vi "Measurement.vi"() -> ()   [LabVIEW 2015]
doc: "Use this template to build a producer/consumer design pattern with events to produce queue items. Use this design pattern instead of the User Interface Event Handler pattern for user interfaces when you want to execute code asynchronously in response to an event without slowing the user interface responsiveness."
uses:
  C:/Program Files (x86)/National Instruments/LabVIEW 2015/examples/Data Communication/Protocols/TCP/TCP Multiple Connections/controls/TCP Multiple Connections State.ctl
panel:
  out "Number  of dev Connected":i32
  in  "Restart":bool
  out "IP Address":string
  out "Waveform_main 2":waveform(sgl)(graph)
  out "CT2":timestamp
  out "USB_DEV2":string
  out "USB_DEV1":string
  out "CT1":timestamp
  out "Waveform_main":waveform(sgl)(graph)
  # "uPower Server V1.0"
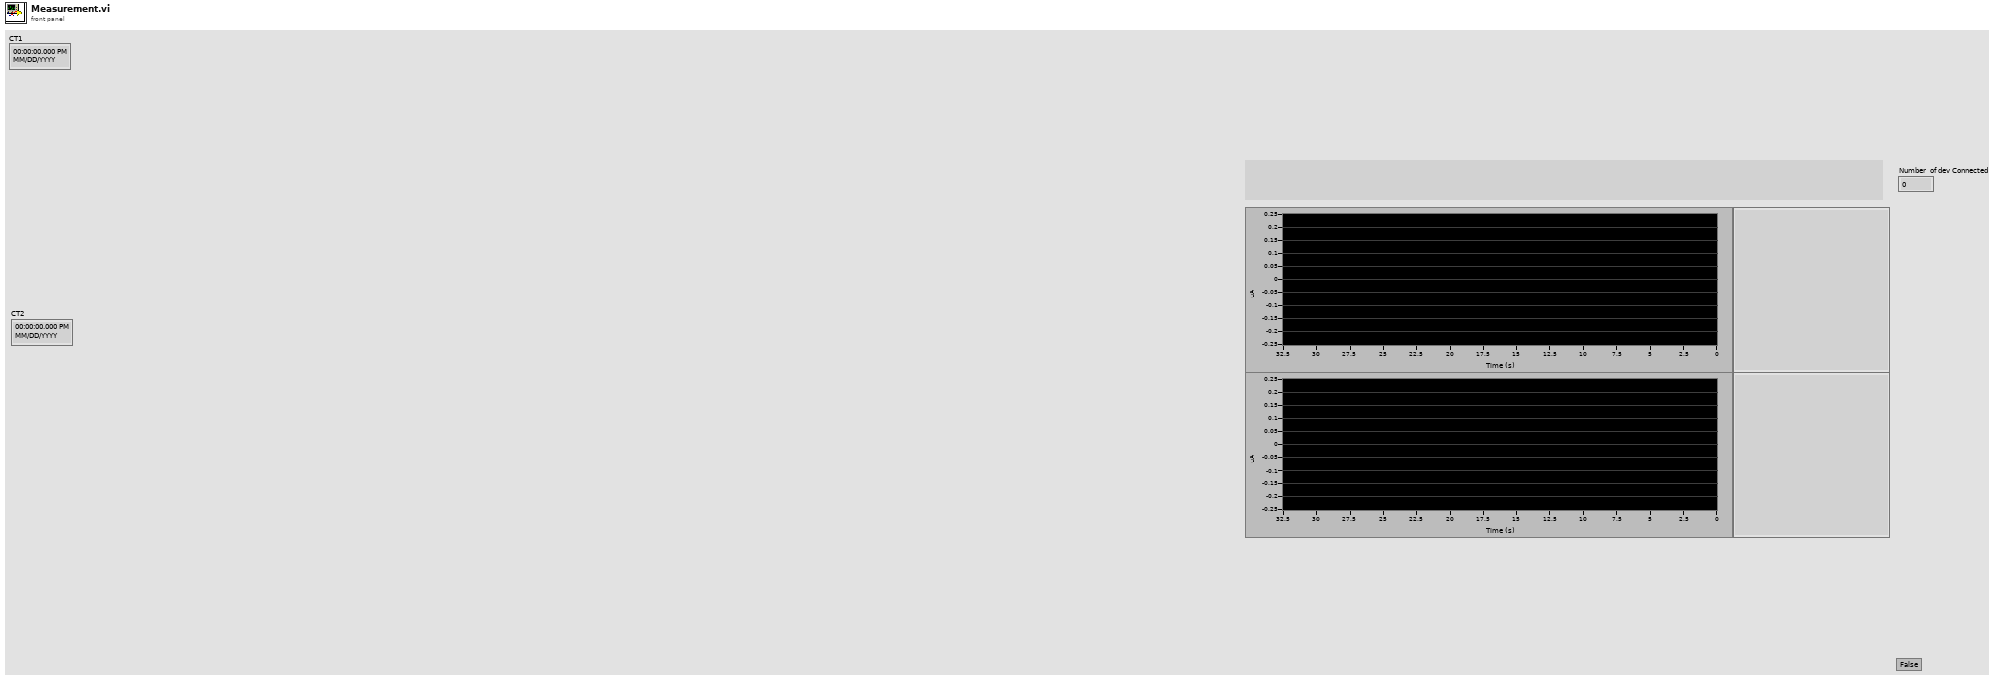
[diagram p1: front panel]
types:
  T1 = typedef "TCP Multiple Connections State.ctl" = enum16{"Initialize", "Status Check", "Measurement", "Return Values to DEV", "Stop"}
  T2 = typedef "uPower_kit.ctl" = cluster{"DEV":string, "BUSY":bool, "VBAT":dbl, "OUTPUT":bool, "LAST_RESULT":dbl, "DURATION":u16, "TRIGGER":bool, "RANGE":string, "Vsource":dbl, "FW":string, "Mode":string}
  T3 = typedef "imagedata.ctl" = cluster{"image type":i32, "image depth":i32, "image":u8[], "mask":u8[], "colors":u32[], "Rectangle":cluster{"left":i16, "top":i16, "right":i16, "bottom":i16}}
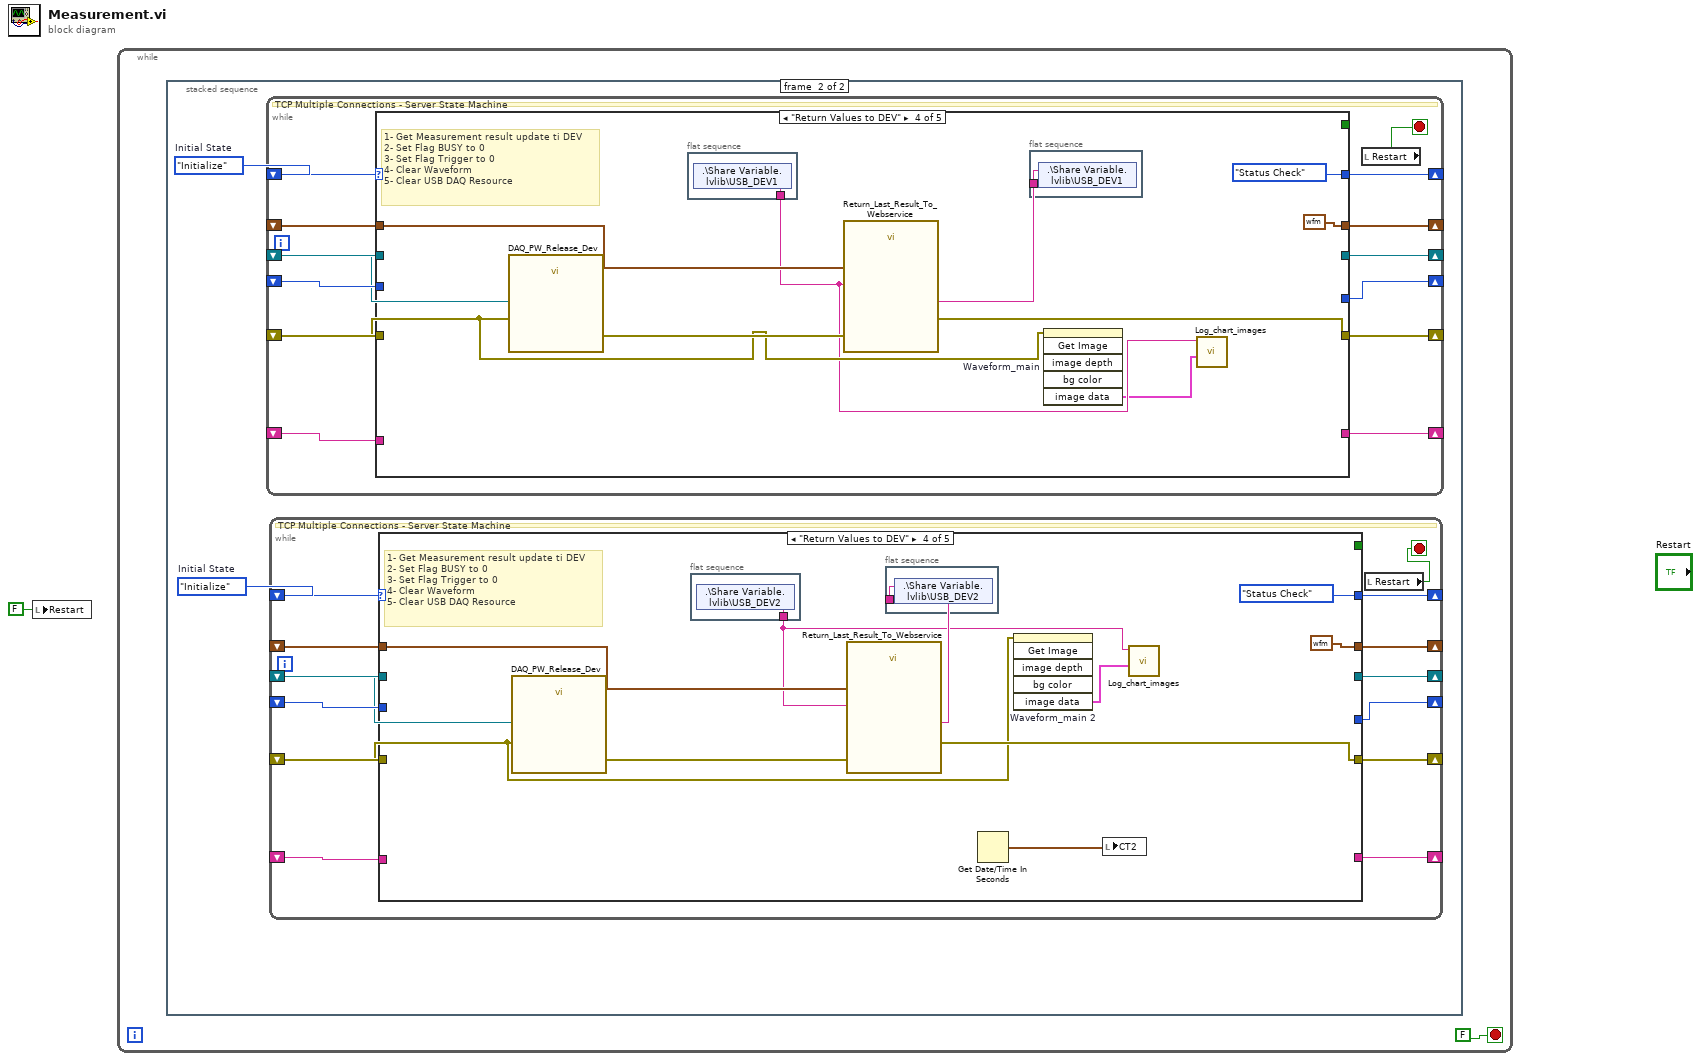
[diagram p0: block diagram]
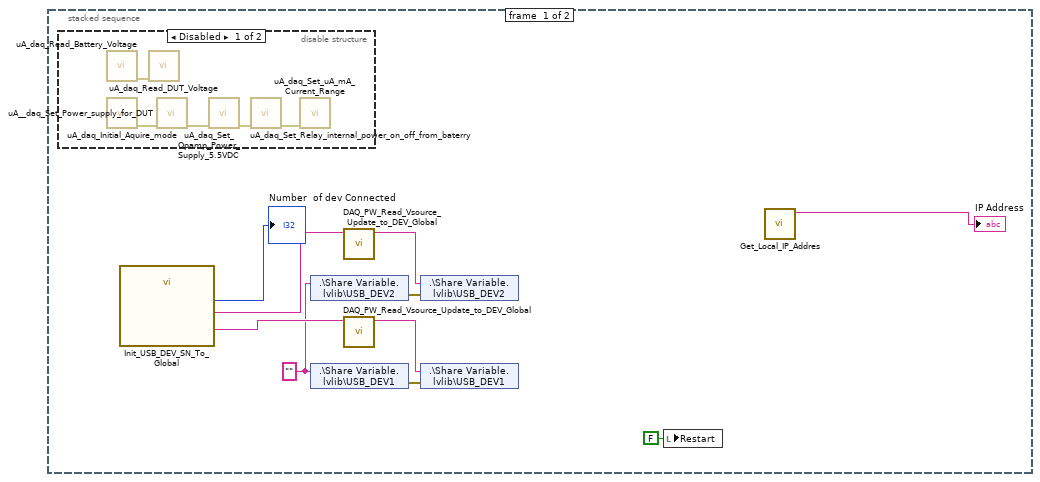
[diagram p2: hidden frame]
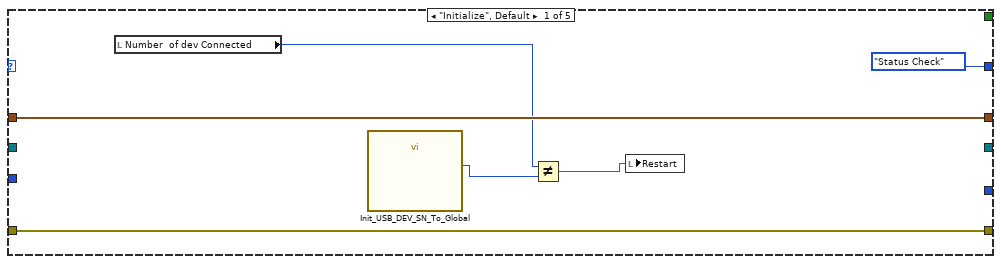
[diagram p4: hidden frame]
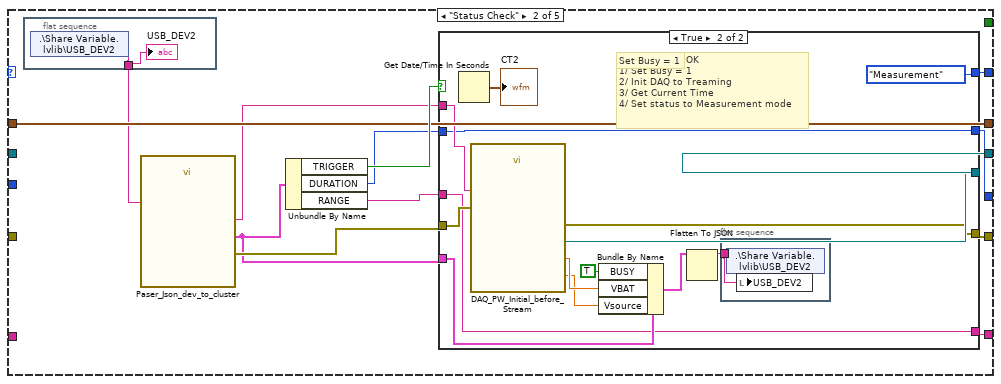
[diagram p5: hidden frame]
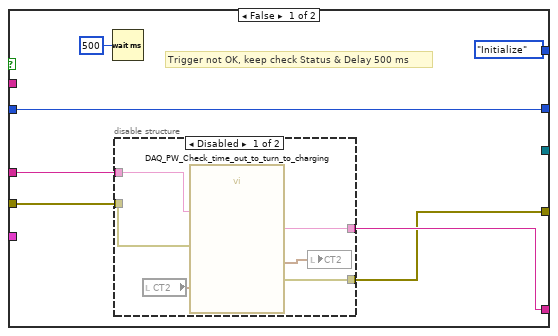
[diagram p6: hidden frame]
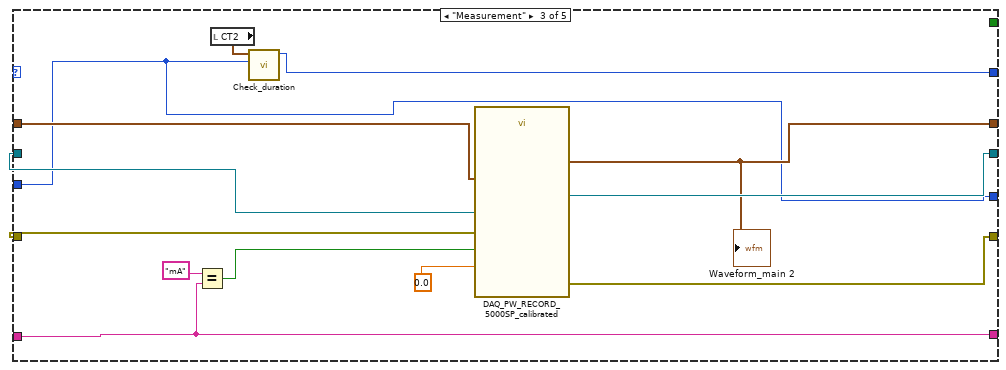
[diagram p8: hidden frame]
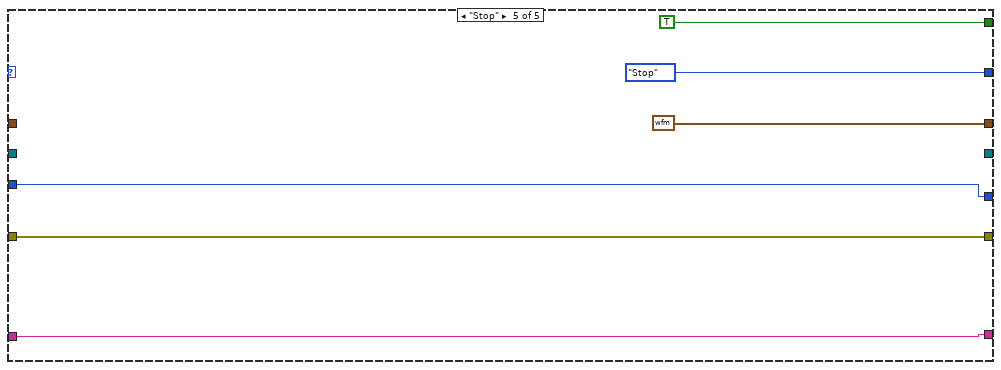
[diagram p9: hidden frame]
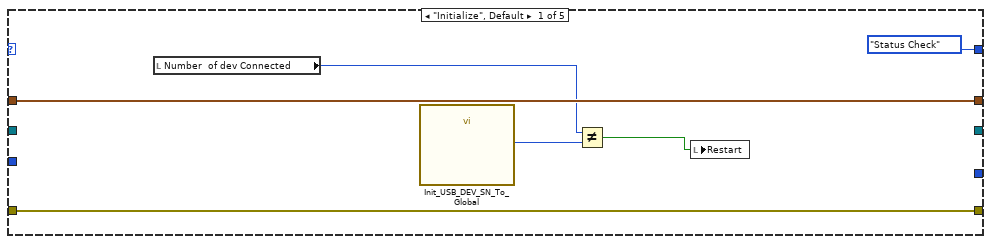
[diagram p10: hidden frame]
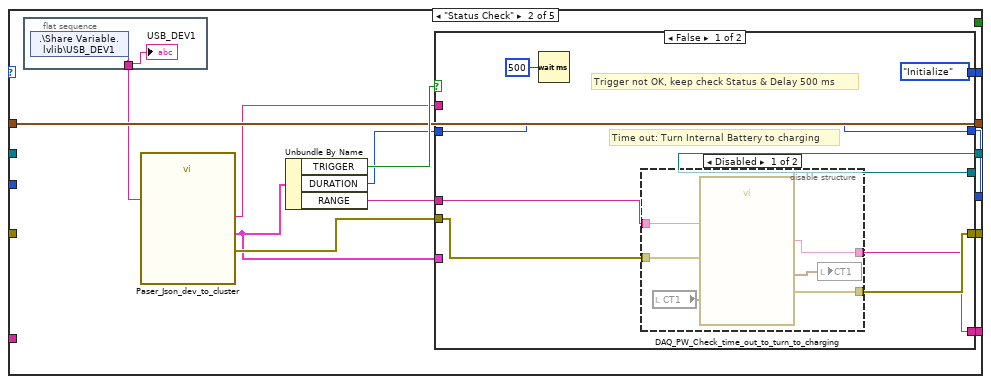
[diagram p11: hidden frame]
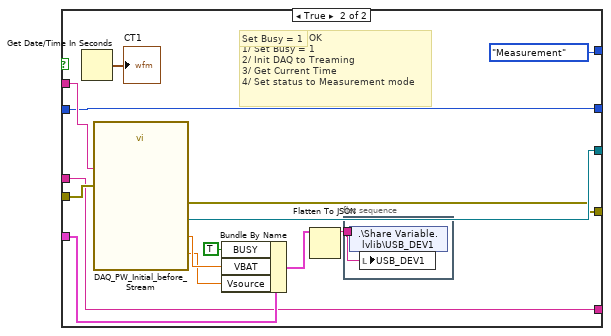
[diagram p13: hidden frame]
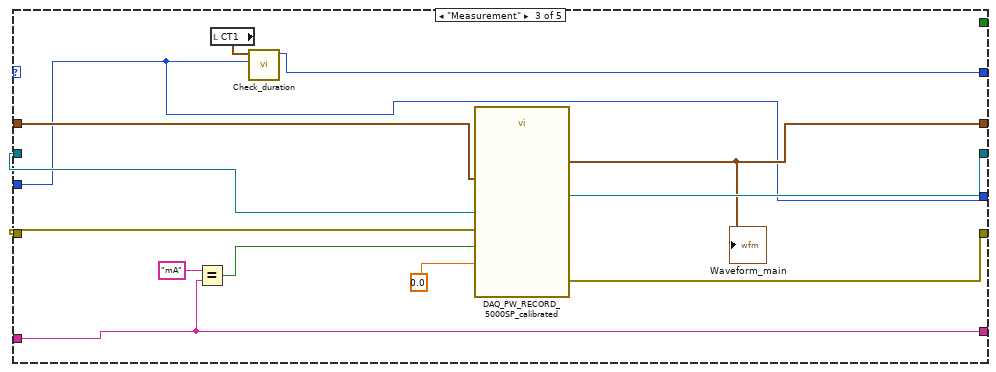
[diagram p14: hidden frame]
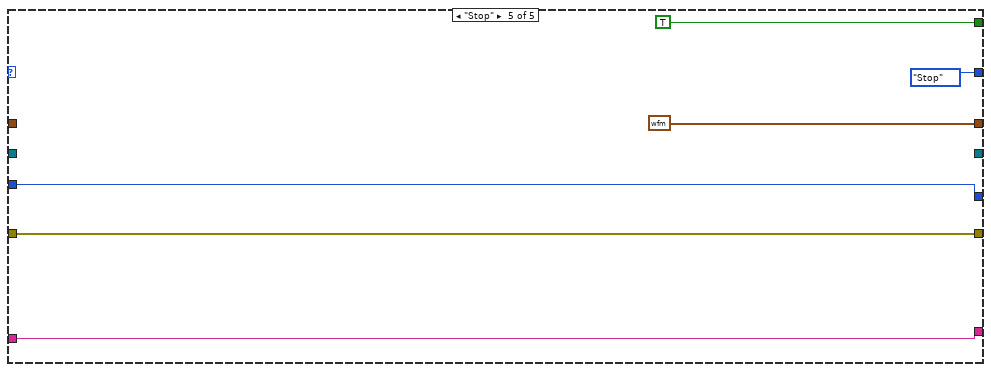
[diagram p15: hidden frame]
diagram:
  n1 = local write "Restart"(FALSE ("Restart")) -> ()
  n2 = while {
    stop <- FALSE stop-if-true
    n3 = stacked-sequence {
      frame #0 {
        w6 = "" ("USB_DEV2")
        n4 = disable-structure shown="Disabled" {
          frame Disabled {
            n5 = call "uA_daq_Read_Battery_Voltage.vi"() -> ("error out"=w13:errorcluster)  [unwired: 10 in, 1 out]
            n6 = call "uA_daq_Initial_Aquire_mode.vi"() -> ("error out"=w14:errorcluster)  [unwired: 10 in, 1 out]
            n7 = call "uA_daq_Read_DUT_Voltage.vi"("error in"=w13) -> ()  [unwired: 9 in, 2 out]
            n8 = call "uA__daq_Set_Power_supply_for_DUT.vi"("error in"=w14) -> ("error out"=w17:errorcluster)  [unwired: 10 in]
            n9 = call "uA_daq_Set_Opamp_Power_Supply_5.5VDC.vi"("error in"=w17) -> ("error out"=w16:errorcluster)  [unwired: 10 in]
            n10 = call "uA_daq_Set_Relay_internal_power_on_off_from_baterry.vi"("error in"=w16) -> ("error out"=w15:errorcluster)  [unwired: 10 in]
            n11 = call "uA_daq_Set_uA_mA_Current_Range.vi"("error in"=w15) -> ()  [unwired: 10 in, 1 out]
          }
          frame Enabled {
          }
        }
        n12 = call "Init_USB_DEV_SN_To_Global.vi"() -> ("Number  of dev Connected"=→"Number  of dev Connected":i32, "USB_DEV_2"=w10:string, "USB_DEV_1"=w12:string)  [unwired: 9 in]
        n13 = shared-variable ".\\Share Variable.lvlib\\USB_DEV2"(w6) -> (error out=w8:errorcluster)  [unwired: 1 in]
        n14 = shared-variable ".\\Share Variable.lvlib\\USB_DEV1"(w6) -> (error out=w7:errorcluster)  [unwired: 1 in]
        n15 = call "DAQ_PW_Read_Vsource_Update_to_DEV_Global.vi"("USB_DEV_1 in"=w10) -> ("USB_DEV_1 out"=w9:string)  [unwired: 10 in]
        n16 = call "DAQ_PW_Read_Vsource_Update_to_DEV_Global.vi"("USB_DEV_1 in"=w12) -> ("USB_DEV_1 out"=w11:string)  [unwired: 10 in]
        n17 = shared-variable ".\\Share Variable.lvlib\\USB_DEV2"(w9, error in=w8) -> ()  [unwired: 1 out]
        n18 = shared-variable ".\\Share Variable.lvlib\\USB_DEV1"(w11, error in=w7) -> ()  [unwired: 1 out]
        n19 = local write "Restart"(FALSE ("Restart")) -> ()
        n20 = call "Get_Local_IP_Addres.vi"() -> ("IP Address"=→"IP Address":string)  [unwired: 11 in]
      }
      frame #1 {
        w18 = TCP_Multiple_Connections_State."Initialize"  # Initial State
        w19 = TCP_Multiple_Connections_State."Initialize"  # Initial State
        n21 = while {
          shift-right: [w124] -> _
          shift-left: w19 -> [w125]
          shift-right: [w121] -> _
          shift-left: _ -> [w120]
          shift-right: [w123] -> _
          shift-left: _ -> [w122]
          shift-right: [w114] -> _
          shift-left: _ -> [w119]
          shift-right: [w117] -> _
          shift-left: _ -> [w118]
          shift-right: [w115] -> _
          shift-left: _ -> [w116]
          stop <- w113 stop-if-true
          # "TCP Multiple Connections - Server State Machine"
          n22 = case shown="\"Return Values to DEV\"" w125 {
            tunnel: [TCP_Multiple_Connections_State."Status Check" ("Initial State") w143 w182 TCP_Multiple_Connections_State."Status Check" ("Initial State") TCP_Multiple_Connections_State."Stop" ("Initial State")] -> w124
            tunnel: [_ _ _ _ TRUE] -> _
            tunnel: [_ w142 w185 _ _] -> w121
            tunnel: [w129 w141 w178 w190 w201] -> w123
            tunnel: w122 -> [w129 _ w179 w189 w201]
            tunnel: w120 -> [_ _ w184 w192 _]
            tunnel: w119 -> [_ _ w176 _ w200]
            tunnel: w118 -> [w130 w139 w181 w194 _]
            tunnel: [w130 w139 w180 waveform(sgl) {"t0"=timestamp(0 s since 1904-01-01), "dt"=1.0, "Y"=[]} ("waveform out") waveform(sgl) {"t0"=timestamp(0 s since 1904-01-01), "dt"=1.0, "Y"=[]} ("waveform out")] -> w117
            tunnel: [_ w135 w177 _ w199] -> w115
            tunnel: w116 -> [_ _ w177 _ w199]
            tunnel: [_ w132 w176 _ w200] -> w114
            frame "Initialize", Default {
              n23 = local read "Number  of dev Connected"() -> (w128:i32)
              n24 = call "Init_USB_DEV_SN_To_Global.vi"() -> ("Number  of dev Connected"=w127:i32)  [unwired: 9 in, 2 out]
              n25 = Not Equal?(x=w128, y=w127) -> (x != y?=w126:bool)
              n26 = local write "Restart"(w126) -> ()
            }
            frame "Status Check" {
              n27 = flat-sequence {
                tunnel: [w145] -> w134
                frame #0 {
                  n28 = shared-variable ".\\Share Variable.lvlib\\USB_DEV1"() -> (w145:string)  [unwired: 1 in, 1 out]
                  "USB_DEV1" <- w145
                }
              }
              n29 = call "Paser_Json_dev_to_cluster.vi"("USB_DEV_IN"=w134) -> ("error out"=w140:errorcluster, "USB_DEV_OUT"=w133:string, "DEV_BUSY"=w138:T2)  [unwired: 8 in]
              n30 = Unbundle By Name(w138) -> ("TRIGGER"=w144:bool, "DURATION"=w137:u16, "RANGE"=w136:string)
              n31 = case shown="False" w144 {
                tunnel: [TCP_Multiple_Connections_State."Initialize" ("Initial State") TCP_Multiple_Connections_State."Measurement" ("Initial State")] -> w143
                tunnel: w133 -> [_ w171]
                tunnel: [_ w169] -> w142
                tunnel: [w147 w164] -> w141
                tunnel: w140 -> [w148 w170]
                tunnel: w138 -> [_ w167]
                tunnel: w137 -> [w150 w162]
                tunnel: w136 -> [w149 w163]
                tunnel: [w150 w162] -> w135
                tunnel: [w146 w163] -> w132
                frame False {
                  # "Time out: Turn Internal Battery to charging"
                  # "Trigger not OK, keep check Status & Delay 500 ms"
                  n32 = Wait (ms)(milliseconds to wait=u32 500) -> ()  [unwired: 1 out]
                  n33 = disable-structure shown="Disabled" {
                    disable-tunnel: w149 -> [w158 _]
                    disable-tunnel: w148 -> [w157 _]
                    disable-tunnel: [w156 _] -> w147
                    disable-tunnel: [w155 _] -> w146
                    frame Disabled {
                      n34 = local read "CT1"() -> (w154:timestamp)
                      n35 = call "DAQ_PW_Check_time_out_to_turn_to_charging.vi"("error in (no error)"=w157, "USB_DEV_Json in"=w158, "CT1_in"=w154) -> ("error in (no error) 2"=w156:errorcluster, "USB_DEV_Json out"=w155:string, "CT1_out"=w153:timestamp)  [unwired: 6 in]
                      n36 = local write "CT1"(w153) -> ()
                    }
                    frame Enabled {
                    }
                  }
                }
                frame True {
                  # "- Trugger = 1 OK\n1/ Set Busy = 1\n2/ Init DAQ to Treaming\n3/ Get Current Time\n4/ Set status to Measurement mode"
                  # "Set Busy = 1"
                  n37 = Get Date/Time In Seconds() -> (seconds since 1Jan1904=→"CT1":timestamp)
                  n38 = call "DAQ_PW_Initial_before_Stream.vi"("error in (no error)"=w170, "USB_DEV_IN"=w171) -> ("error out"=w164:errorcluster, "Vbat"=w160:dbl, "Vsource"=w159:dbl, "Refnum out"=w169:refnum<k21>)  [unwired: 6 in]
                  n39 = Bundle By Name(cluster=w167, "BUSY"=TRUE, "VBAT"=w160, "Vsource"=w159) -> (w165:T2)
                  n40 = Flatten To JSON(anything=w165) -> (JSON string=w161:string)  [unwired: 2 in, 1 out]
                  n41 = flat-sequence {
                    tunnel: w161 -> [w173]
                    frame #0 {
                      n42 = shared-variable ".\\Share Variable.lvlib\\USB_DEV1"(w173) -> ()  [unwired: 1 in, 1 out]
                      n43 = local write "USB_DEV1"(w173) -> ()
                    }
                  }
                }
              }
            }
            frame "Measurement" {
              n44 = Equal?(x="mA", y=w176) -> (x = y?=w174:bool)
              n45 = local read "CT1"() -> (w183:timestamp)
              n46 = call "Check_duration.vi"("Duration"=w177, "CT1"=w183) -> ("Initial State"=w182:T1)  [unwired: 9 in]
              n47 = call "DAQ_PW_RECORD_5000SP_calibrated.vi"("waveform in"=w181, "error in"=w179, "MA/UA"=w174, "calibration"=0.0, "DAQ in"=w184) -> ("error out"=w178:errorcluster, "waveform out 2"=w180:waveform(sgl), "DAQ out"=w185:refnum<k21>)  [unwired: 4 in]
              "Waveform_main" <- w180
            }
            frame "Return Values to DEV" {
              # "1- Get Measurement result update ti DEV\n2- Set Flag BUSY to 0\n3- Set Flag Trigger to 0\n4- Clear Waveform\n5- Clear USB DAQ Resource"
              n48 = call "DAQ_PW_Release_Dev.vi"("error in (no error)"=w189, "Refnum in"=w192) -> ("error out"=w191:errorcluster)  [unwired: 9 in]
              n49 = flat-sequence {
                tunnel: [w197] -> w188
                frame #0 {
                  n50 = shared-variable ".\\Share Variable.lvlib\\USB_DEV1"() -> (w197:string)  [unwired: 1 in, 1 out]
                }
              }
              n51 = call "Return_Last_Result_To_Webservice.vi"("error in (no error)"=w191, "String"=w188, "waveform in"=w194) -> ("error out"=w190:errorcluster, "JSON string"=w193:string)  [unwired: 7 in]
              n52 = flat-sequence {
                tunnel: w193 -> [w198]
                frame #0 {
                  n53 = shared-variable ".\\Share Variable.lvlib\\USB_DEV1"(w198) -> ()  [unwired: 1 in, 1 out]
                }
              }
              n54 = invoke on="Waveform_main" class="WFGraph (strict)" method="Get Image"(error in=w189) -> ("image data"=w187:T3)  [unwired: 5 in, 5 out]
              n55 = call "Log_chart_images.vi"("image data"=w187, "JSON DEV"=w188) -> ()  [unwired: 9 in, 1 out]
            }
            frame "Stop" {
            }
          }
          n56 = local read "Restart"() -> (w113:bool)
        }
        n57 = while {
          shift-right: [w31] -> _
          shift-left: w18 -> [w32]
          shift-right: [w28] -> _
          shift-left: _ -> [w27]
          shift-right: [w30] -> _
          shift-left: _ -> [w29]
          shift-right: [w21] -> _
          shift-left: _ -> [w26]
          shift-right: [w24] -> _
          shift-left: _ -> [w25]
          shift-right: [w22] -> _
          shift-left: _ -> [w23]
          stop <- w20 stop-if-true
          # "TCP Multiple Connections - Server State Machine"
          n58 = case shown="\"Return Values to DEV\"" w32 {
            tunnel: [TCP_Multiple_Connections_State."Status Check" ("Initial State") w50 w89 TCP_Multiple_Connections_State."Status Check" ("Initial State") TCP_Multiple_Connections_State."Stop" ("Initial State")] -> w31
            tunnel: [_ _ _ _ TRUE] -> _
            tunnel: [_ w49 w92 _ _] -> w28
            tunnel: [w36 w48 w85 w98 w109] -> w30
            tunnel: w29 -> [w36 _ w86 w95 w109]
            tunnel: w27 -> [_ _ w91 w100 _]
            tunnel: w26 -> [_ _ w83 _ w108]
            tunnel: w25 -> [w37 w46 w88 w102 _]
            tunnel: [w37 w46 w87 waveform(sgl) {"t0"=timestamp(0 s since 1904-01-01), "dt"=1.0, "Y"=[]} ("waveform out") waveform(sgl) {"t0"=timestamp(0 s since 1904-01-01), "dt"=1.0, "Y"=[]} ("waveform out")] -> w24
            tunnel: [_ w42 w84 _ w107] -> w22
            tunnel: w23 -> [_ _ w84 _ w107]
            tunnel: [_ w39 w83 _ w108] -> w21
            frame "Initialize", Default {
              n59 = local read "Number  of dev Connected"() -> (w34:i32)
              n60 = call "Init_USB_DEV_SN_To_Global.vi"() -> ("Number  of dev Connected"=w35:i32)  [unwired: 9 in, 2 out]
              n61 = Not Equal?(x=w34, y=w35) -> (x != y?=w33:bool)
              n62 = local write "Restart"(w33) -> ()
            }
            frame "Status Check" {
              n63 = flat-sequence {
                tunnel: [w52] -> w41
                frame #0 {
                  n64 = shared-variable ".\\Share Variable.lvlib\\USB_DEV2"() -> (w52:string)  [unwired: 1 in, 1 out]
                  "USB_DEV2" <- w52
                }
              }
              n65 = call "Paser_Json_dev_to_cluster.vi"("USB_DEV_IN"=w41) -> ("error out"=w47:errorcluster, "USB_DEV_OUT"=w40:string, "DEV_BUSY"=w45:T2)  [unwired: 8 in]
              n66 = Unbundle By Name(w45) -> ("TRIGGER"=w51:bool, "DURATION"=w44:u16, "RANGE"=w43:string)
              n67 = case shown="True" w51 {
                tunnel: [TCP_Multiple_Connections_State."Initialize" ("Initial State") TCP_Multiple_Connections_State."Measurement" ("Initial State")] -> w50
                tunnel: w40 -> [_ w78]
                tunnel: [_ w76] -> w49
                tunnel: [w53 w71] -> w48
                tunnel: w47 -> [w54 w77]
                tunnel: w45 -> [_ w74]
                tunnel: w44 -> [w57 w69]
                tunnel: w43 -> [w56 w70]
                tunnel: [w57 w69] -> w42
                tunnel: [w55 w70] -> w39
                frame False {
                  # "Trigger not OK, keep check Status & Delay 500 ms"
                  n68 = Wait (ms)(milliseconds to wait=u32 500) -> ()  [unwired: 1 out]
                  n69 = disable-structure shown="Disabled" {
                    disable-tunnel: w56 -> [w63 _]
                    disable-tunnel: [w62 _] -> w55
                    disable-tunnel: w54 -> [w61 _]
                    disable-tunnel: [w60 _] -> w53
                    frame Disabled {
                      n70 = local read "CT2"() -> (w64:timestamp)
                      n71 = call "DAQ_PW_Check_time_out_to_turn_to_charging.vi"("error in (no error)"=w61, "USB_DEV_Json in"=w63, "CT1_in"=w64) -> ("error in (no error) 2"=w60:errorcluster, "USB_DEV_Json out"=w62:string, "CT1_out"=w65:timestamp)  [unwired: 6 in]
                      n72 = local write "CT2"(w65) -> ()
                    }
                    frame Enabled {
                    }
                  }
                }
                frame True {
                  # "- Trugger = 1 OK\n1/ Set Busy = 1\n2/ Init DAQ to Treaming\n3/ Get Current Time\n4/ Set status to Measurement mode"
                  # "Set Busy = 1"
                  n73 = Get Date/Time In Seconds() -> (seconds since 1Jan1904=→"CT2":timestamp)
                  n74 = call "DAQ_PW_Initial_before_Stream.vi"("error in (no error)"=w77, "USB_DEV_IN"=w78) -> ("error out"=w71:errorcluster, "Vbat"=w67:dbl, "Vsource"=w66:dbl, "Refnum out"=w76:refnum<k21>)  [unwired: 6 in]
                  n75 = Bundle By Name(cluster=w74, "BUSY"=TRUE, "VBAT"=w67, "Vsource"=w66) -> (w72:T2)
                  n76 = Flatten To JSON(anything=w72) -> (JSON string=w68:string)  [unwired: 2 in, 1 out]
                  n77 = flat-sequence {
                    tunnel: w68 -> [w80]
                    frame #0 {
                      n78 = shared-variable ".\\Share Variable.lvlib\\USB_DEV2"(w80) -> ()  [unwired: 1 in, 1 out]
                      n79 = local write "USB_DEV2"(w80) -> ()
                    }
                  }
                }
              }
            }
            frame "Measurement" {
              n80 = Equal?(x="mA", y=w83) -> (x = y?=w81:bool)
              n81 = local read "CT2"() -> (w90:timestamp)
              n82 = call "Check_duration.vi"("Duration"=w84, "CT1"=w90) -> ("Initial State"=w89:T1)  [unwired: 9 in]
              n83 = call "DAQ_PW_RECORD_5000SP_calibrated.vi"("waveform in"=w88, "error in"=w86, "MA/UA"=w81, "calibration"=0.0, "DAQ in"=w91) -> ("error out"=w85:errorcluster, "waveform out 2"=w87:waveform(sgl), "DAQ out"=w92:refnum<k21>)  [unwired: 4 in]
              "Waveform_main 2" <- w87
            }
            frame "Return Values to DEV" {
              # "1- Get Measurement result update ti DEV\n2- Set Flag BUSY to 0\n3- Set Flag Trigger to 0\n4- Clear Waveform\n5- Clear USB DAQ Resource"
              n84 = call "DAQ_PW_Release_Dev.vi"("error in (no error)"=w95, "Refnum in"=w100) -> ("error out"=w99:errorcluster)  [unwired: 9 in]
              n85 = flat-sequence {
                tunnel: [w105] -> w94
                frame #0 {
                  n86 = shared-variable ".\\Share Variable.lvlib\\USB_DEV2"() -> (w105:string)  [unwired: 1 in, 1 out]
                }
              }
              n87 = call "Return_Last_Result_To_Webservice.vi"("error in (no error)"=w99, "String"=w94, "waveform in"=w102) -> ("error out"=w98:errorcluster, "JSON string"=w101:string)  [unwired: 7 in]
              n88 = flat-sequence {
                tunnel: w101 -> [w106]
                frame #0 {
                  n89 = shared-variable ".\\Share Variable.lvlib\\USB_DEV2"(w106) -> ()  [unwired: 1 in, 1 out]
                }
              }
              n90 = Get Date/Time In Seconds() -> (seconds since 1Jan1904=w97:timestamp)
              n91 = invoke on="Waveform_main 2" class="WFGraph (strict)" method="Get Image"(error in=w95) -> ("image data"=w96:T3)  [unwired: 5 in, 5 out]
              n92 = local write "CT2"(w97) -> ()
              n93 = call "Log_chart_images.vi"("image data"=w96, "JSON DEV"=w94) -> ()  [unwired: 9 in, 1 out]
            }
            frame "Stop" {
            }
          }
          n94 = local read "Restart"() -> (w20:bool)
        }
      }
    }
  }
